vi "Decode Text.vi"(4 "error in":errorcluster, 6 "Encoded String":string, 7 "Text Ref":refnum<vi>) -> (0 "error out":errorcluster, 3 "dup Text Ref":refnum<vi>)   [LabVIEW 2018]
doc: "Reads an HTML-like string with attribute spefifications for:\nFont name, size, color, bold, italic, underline, & strikeout, and\nputs the value with attributes into the referenced string."
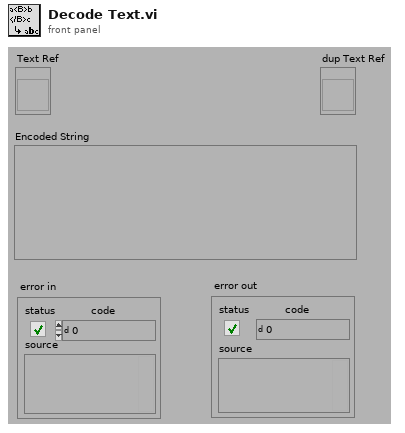
[diagram p1: front panel]
types:
  T1 = typedef "LVFontTypeDef.ctl" = cluster{"Font Name":string, "Size":u16, "Bold":bool, "Italic":bool, "Underline":bool, "Strikeout":bool, "Color":u32}
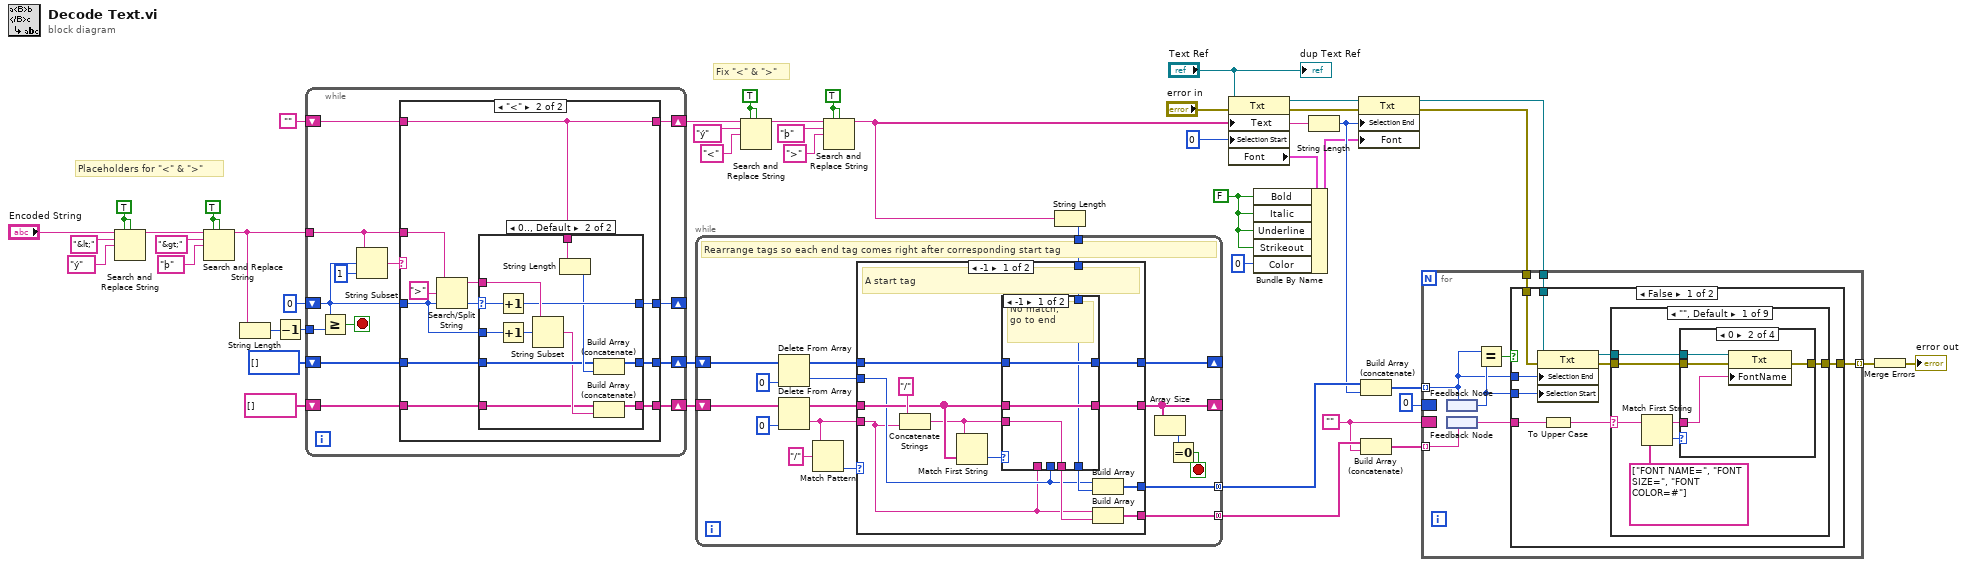
[diagram p0: block diagram]
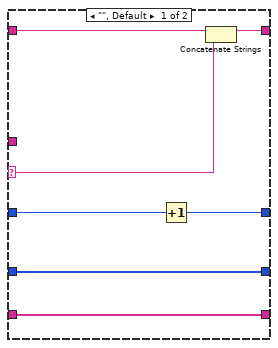
[diagram p2: hidden frame]
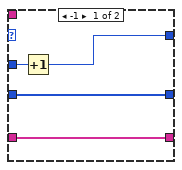
[diagram p3: hidden frame]
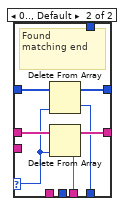
[diagram p4: hidden frame]
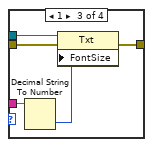
[diagram p7: hidden frame]
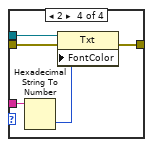
[diagram p8: hidden frame]
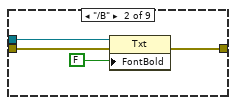
[diagram p9: hidden frame]
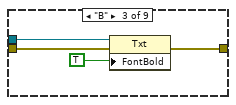
[diagram p10: hidden frame]
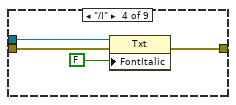
[diagram p11: hidden frame]
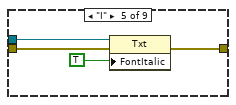
[diagram p12: hidden frame]
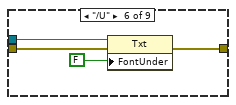
[diagram p13: hidden frame]
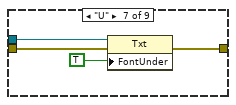
[diagram p14: hidden frame]
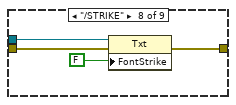
[diagram p15: hidden frame]
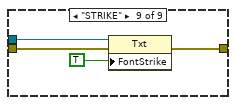
[diagram p16: hidden frame]
diagram:
  w22 = FALSE ("Bold")
  w29 = TRUE ("replace all? (F)")
  w32 = TRUE ("replace all? (F)")
  w36 = TRUE ("replace all? (F)")
  w39 = TRUE ("replace all? (F)")
  w9 = ""
  # "Fix \"<\" & \">\""
  # "Placeholders for \"<\" & \">\""
  n1 = Search and Replace String(replace all?=w39, case sensitive?=w39, input string="Encoded String", search string="&lt;", replace string="ý" ("replace string (\"\")")) -> (result string=w34:string)  [unwired: 3 in, 3 out]
  n2 = Search and Replace String(replace all?=w36, case sensitive?=w36, input string=w34, search string="&gt;", replace string="þ" ("replace string (\"\")")) -> (result string=w26:string)  [unwired: 3 in, 3 out]
  n3 = String Length(string=w26) -> (length=w46:i32)
  n4 = Decrement(x=w46) -> (x-1=w45:i32)
  n5 = while {
    tunnel: w26 -> [w54]
    shift-right: [w58] -> _
    shift-left: 0 ("length (rest)") -> [w56]
    tunnel: w45 -> [w57]
    shift-right: [w52] -> w8
    shift-left: "" -> [w53]
    shift-right: [w51] -> w17
    shift-left: i32[] [] -> [w50]
    shift-right: [w49] -> w16
    shift-left: string[] [] -> [w48]
    stop <- w55 stop-if-true
    n6 = Greater Or Equal?(x=w56, y=w57) -> (x >= y?=w55:bool)
    n7 = String Subset(string=w54, offset (0)=w56, length (rest)=1 ("length (rest)")) -> (substring=w59:string)
    n8 = case shown="\"<\"" w59 {
      selector: w59 -> [w67 _]
      tunnel: w56 -> [w66 w74]
      tunnel: [w65 w73] -> w58
      tunnel: w54 -> [_ w76]
      tunnel: w53 -> [w64 w72]
      tunnel: [w63 w72] -> w52
      tunnel: [w62 w71] -> w51
      tunnel: w50 -> [w62 w70]
      tunnel: [w61 w69] -> w49
      tunnel: w48 -> [w61 w68]
      frame "", Default {
        n9 = Increment(x=w66) -> (x+1=w65:i32)
        n10 = Concatenate Strings(w64, w67) -> (w63:string)
      }
      frame "<" {
        n11 = Search/Split String(string=w76, search string/char (-)=">", offset (0)=w74) -> (substring before match=w75:string, offset of match=w77:i32)  [unwired: 1 out]
        n12 = case shown="0.., Default" w77 {
          selector: w77 -> [_ w93]
          tunnel: w75 -> [_ w92]
          tunnel: w74 -> [w82 w91]
          tunnel: [w81 w90] -> w73
          tunnel: w72 -> [_ w89]
          tunnel: [w80 w86] -> w71
          tunnel: w70 -> [w80 w87]
          tunnel: [w79 w85] -> w69
          tunnel: w68 -> [w79 w83]
          frame -1 {
            n13 = Increment(x=w82) -> (x+1=w81:i32)
          }
          frame 0.., Default {
            n14 = Increment(x=w93) -> (x+1=w90:i32)
            n15 = Increment(x=w91) -> (x+1=w94:i32)
            n16 = String Subset(string=w92, offset (0)=w94) -> (substring=w84:string)  [unwired: 1 in]
            n17 = String Length(string=w89) -> (length=w88:i32)
            n18 = Build Array (concatenate)(w87, w88) -> (w86:i32[])
            n19 = Build Array (concatenate)(w83, w84) -> (w85:string[])
          }
        }
      }
    }
  }
  n20 = Search and Replace String(replace all?=w32, case sensitive?=w32, input string=w8, search string="ý", replace string="<" ("replace string (\"\")")) -> (result string=w27:string)  [unwired: 3 in, 3 out]
  n21 = Search and Replace String(replace all?=w29, case sensitive?=w29, input string=w27, search string="þ", replace string=">" ("replace string (\"\")")) -> (result string=w6:string)  [unwired: 3 in, 3 out]
  n22 = String Length(string=w6) -> (length=w7:i32)
  n23 = while {
    shift-right: [w99] -> _
    shift-left: w17 -> [w111]
    shift-right: [w98] -> _
    shift-left: w16 -> [w108]
    tunnel: [w102] -> w15 mode=concatenating
    tunnel: [w100] -> w13 mode=concatenating
    tunnel: w7 -> [w95]
    stop <- w96 stop-if-true
    # "Rearrange tags so each end tag comes right after corresponding start tag"
    n24 = Delete From Array(array=w111, index=0) -> (deleted portion=w105:i32, array with subset deleted=w104:i32[])  [unwired: 1 in]
    n25 = Delete From Array(array=w108, index=0) -> (deleted portion=w101:string, array with subset deleted=w103:string[])  [unwired: 1 in]
    n26 = Match Pattern(string=w101, regular expression="/" ("search string/char (-)")) -> (offset past match=w106:i32)  [unwired: 1 in, 3 out]
    n27 = case shown="-1" w106 {
      tunnel: w105 -> [w116 w137]
      tunnel: w104 -> [w121 w140]
      tunnel: w103 -> [w123 w142]
      tunnel: [w114 w138] -> w102
      tunnel: w101 -> [w115 w141]
      tunnel: [w113 w139] -> w100
      tunnel: [w122 w142] -> w98
      tunnel: [w120 w140] -> w99
      tunnel: w95 -> [w112 _]
      frame -1 {
        # "A start tag"
        n28 = Concatenate Strings("/" ("string"), w115) -> (w119:string)
        n29 = Match First String(2:w123, 3:w119) -> (0:w124:i32)  [unwired: 1 out]
        n30 = case shown="-1" w124 {
          selector: w124 -> [_ w132]
          tunnel: w123 -> [w128 w136]
          tunnel: [w128 w135] -> w122
          tunnel: w121 -> [w129 w134]
          tunnel: [w129 w133] -> w120
          tunnel: w119 -> [w127 _]
          tunnel: [w126 w131] -> w118
          tunnel: [w127 w130] -> w117
          tunnel: w116 -> [_ _]
          tunnel: w115 -> [_ _]
          tunnel: w112 -> [w126 _]
          frame -1 {
            # "No match,\ngo to end"
          }
          frame 0.., Default {
            # "Found\nmatching end"
            n31 = Delete From Array(array=w134, index=w132) -> (deleted portion=w131:i32, array with subset deleted=w133:i32[])  [unwired: 1 in]
            n32 = Delete From Array(array=w136, index=w132) -> (deleted portion=w130:string, array with subset deleted=w135:string[])  [unwired: 1 in]
          }
        }
        n33 = Build Array(w116, w118) -> (w114:i32[])
        n34 = Build Array(w115, w117) -> (w113:string[])
      }
      frame 0.., Default {
        # "An end tag.\npass it through"
        n35 = Build Array(w137) -> (w138:i32[])
        n36 = Build Array(w141) -> (w139:string[])
      }
    }
    n37 = Array Size(array=w98) -> (size(s)=w97:i32)
    n38 = Equal To 0?(x=w97) -> (x = 0?=w96:bool)
  }
  n39 = property on="Property Node" class="Txt"(reference="Text Ref", error in="error in", "Text"=w6, "Selection Start"=u32 0 ("Text.Selection:Start")) -> (reference out=w42:refnum<vi>, error out=w41:errorcluster, "Font"=w20:T1)
  n40 = Bundle By Name(cluster=w20, "Bold"=w22, "Italic"=w22, "Underline"=w22, "Strikeout"=w22, "Color"=u32 0) -> (w5:T1)
  n41 = String Length(string=w6) -> (length=w14:i32)
  n42 = property on="Property Node" class="Txt"(reference=w42, error in=w41, "Selection End"=w14, "Font"=w5) -> (reference out=w24:refnum<vi>, error out=w25:errorcluster)
  n43 = Build Array (concatenate)(w15, w14) -> (w12:i32[])
  n44 = Build Array (concatenate)(w13, w9) -> (w10:string[])
  n45 = for {
    tunnel: w24 -> [w150]
    tunnel: w25 -> [w149]
    tunnel: [w148] -> w23 mode=indexing
    border: 0 -> [_]
    tunnel: w12 -> [w143] mode=indexing
    tunnel: w10 -> [w146] mode=indexing
    border: w9 -> [_]
    n46 = feedback #1() -> (w144:i32)
    n47 = feedback-in #1(w143) -> ()
    n48 = feedback #2() -> (w145:string)
    n49 = feedback-in #2(w146) -> ()
    n50 = Equal?(x=w143, y=w144) -> (x = y?=w147:bool)
    n51 = case shown="False" w147 {
      tunnel: w150 -> [w158 _]
      tunnel: w149 -> [w156 w214]
      tunnel: [w154 w214] -> w148
      tunnel: w145 -> [w153 _]
      tunnel: w143 -> [w152 _]
      tunnel: w144 -> [w151 _]
      frame False {
        n52 = property on="Property Node" class="Txt"(reference=w158, error in=w156, "Selection End"=w152, "Selection Start"=w151) -> (reference out=w159:refnum<vi>, error out=w155:errorcluster)
        n53 = To Upper Case(1:w153) -> (0:w157:string)
        n54 = case shown="\"\", Default" w157 {
          selector: w157 -> [w166 _ _ _ _ _ _ _ _]
          tunnel: w159 -> [w163 w185 w189 w193 w197 w201 w205 w209 w213]
          tunnel: w155 -> [w162 w184 w188 w192 w196 w200 w204 w208 w212]
          tunnel: [w161 w183 w187 w191 w195 w199 w203 w207 w211] -> w154
          frame "", Default {
            n55 = Match First String(2:string[] ["FONT NAME=", "FONT SIZE=", "FONT COLOR=#"], 3:w166) -> (0:w165:i32, 1:w164:string)
            n56 = case shown="0" w165 {
              tunnel: w164 -> [_ w168 w175 w180]
              tunnel: w163 -> [_ w171 w176 w181]
              tunnel: w162 -> [w167 w170 w174 w179]
              tunnel: [w167 w169 w173 w178] -> w161
              frame -1, Default {
              }
              frame 0 {
                n57 = property on="Property Node" class="Txt"(reference=w171, error in=w170, "FontName"=w168) -> (error out=w169:errorcluster)  [unwired: 1 out]
              }
              frame 1 {
                n58 = Decimal String To Number(string=w175) -> (number=w172:i32)  [unwired: 2 in, 1 out]
                n59 = property on="Property Node" class="Txt"(reference=w176, error in=w174, "FontSize"=w172) -> (error out=w173:errorcluster)  [unwired: 1 out]
              }
              frame 2 {
                n60 = Hexadecimal String To Number(string=w180) -> (number=w177:u32)  [unwired: 2 in, 1 out]
                n61 = property on="Property Node" class="Txt"(reference=w181, error in=w179, "FontColor"=w177) -> (error out=w178:errorcluster)  [unwired: 1 out]
              }
            }
          }
          frame "/B" {
            n62 = property on="Property Node" class="Txt"(reference=w185, error in=w184, "FontBold"=FALSE ("Text.Font:Bold")) -> (error out=w183:errorcluster)  [unwired: 1 out]
          }
          frame "B" {
            n63 = property on="Property Node" class="Txt"(reference=w189, error in=w188, "FontBold"=TRUE ("Text.Font:Bold")) -> (error out=w187:errorcluster)  [unwired: 1 out]
          }
          frame "/I" {
            n64 = property on="Property Node" class="Txt"(reference=w193, error in=w192, "FontItalic"=FALSE ("Text.Font:Bold")) -> (error out=w191:errorcluster)  [unwired: 1 out]
          }
          frame "I" {
            n65 = property on="Property Node" class="Txt"(reference=w197, error in=w196, "FontItalic"=TRUE ("Text.Font:Bold")) -> (error out=w195:errorcluster)  [unwired: 1 out]
          }
          frame "/U" {
            n66 = property on="Property Node" class="Txt"(reference=w201, error in=w200, "FontUnder"=FALSE ("Text.Font:Bold")) -> (error out=w199:errorcluster)  [unwired: 1 out]
          }
          frame "U" {
            n67 = property on="Property Node" class="Txt"(reference=w205, error in=w204, "FontUnder"=TRUE ("Text.Font:Bold")) -> (error out=w203:errorcluster)  [unwired: 1 out]
          }
          frame "/STRIKE" {
            n68 = property on="Property Node" class="Txt"(reference=w209, error in=w208, "FontStrike"=FALSE ("Text.Font:Bold")) -> (error out=w207:errorcluster)  [unwired: 1 out]
          }
          frame "STRIKE" {
            n69 = property on="Property Node" class="Txt"(reference=w213, error in=w212, "FontStrike"=TRUE ("Text.Font:Bold")) -> (error out=w211:errorcluster)  [unwired: 1 out]
          }
        }
      }
      frame True {
        # "Don't mess with 0-length selection at end: It will affect the whole string"
      }
    }
  }
  n70 = Merge Errors(w23) -> (→"error out":errorcluster)
  "dup Text Ref" <- "Text Ref"
